vi "ActionVIDebug.vi"(11 "CompiledSettings":T1 {"Result Ch Data Refs" format="%.0x"; "Parameter Block Data Refs"."Data Reference" format="%.0x"}) -> ()   [LabVIEW 2020, in "Waveform-Processing-Custom-Device System Explorer.lvlib"]
uses:
  Waveform-Processing-Custom-Device System Explorer.lvlib
  Shared/CompiledSettings.ctl
  <vilib>/NI VeriStand/Custom Device API/Block Data Reference.ctl
  <vilib>/NI VeriStand/Custom Device API/Data Reference.ctl
  <vilib>/NI VeriStand/Custom Device API/Waveform Data Reference.ctl
  <vilib>/NI VeriStand/Custom Device API/Custom Device API.lvlib
  Shared/Waveform-Processing-Custom-Device Shared.lvlib
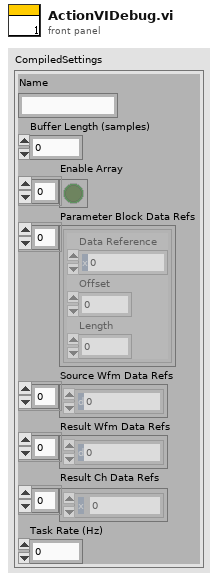
[diagram p1: front panel]
types:
  T1 = typedef "Waveform-Processing-Custom-Device Shared.lvlib/CompiledSettings.ctl" = cluster{"Name":string, "Buffer Length (samples)":u32, "Enable Array":bool[], "Parameter Block Data Refs":T2[], "Source Wfm Data Refs":T4[], "Result Wfm Data Refs":T4[], "Result Ch Data Refs":T3[], "Task Rate (Hz)":dbl}
  T2 = typedef "Custom Device API.lvlib/Block Data Reference.ctl" = cluster{"Data Reference":T3, "Offset":u64, "Length":u64}
  T3 = typedef "Custom Device API.lvlib/Data Reference.ctl" = i32
  T4 = typedef "Custom Device API.lvlib/Waveform Data Reference.ctl" = i32
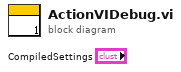
[diagram p0: block diagram]
diagram:
